vi "Test Cryo-Con Read.vi"() -> ()   [LabVIEW 2016]
panel:
  out "data string":string
  out "Temperature":dbl format="%.5f"
  in  "VISA Resource Name":refnum<visa-resource-name>
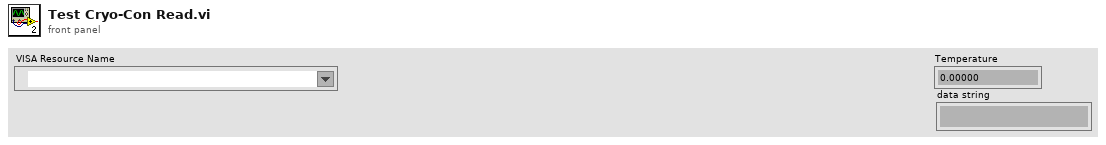
[diagram p1: front panel]
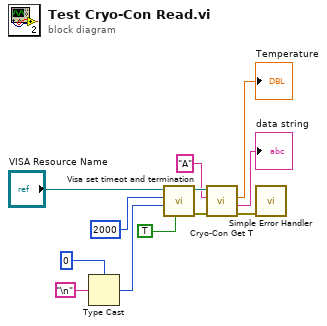
[diagram p0: block diagram]
diagram:
  n1 = Type Cast(type=u8 0, x="\n") -> (*(type *) &x=w3:u8)
  n2 = call "Visa set timeot and termination.vi"("Termination Character Enable"=TRUE, "Termination Character"=w3, "Timeout Value"=u32 2000, "VISA resource name"="VISA Resource Name") -> ("error out"=w2:errorcluster, "VISA resource name out"=w8:refnum<visa-resource-name>)  [unwired: 3 in, 3 out]
  n3 = call "Cryo-Con Get T.vi"("error in (no error)"=w2, "Channel"="A", "VISA Resource Name"=w8) -> ("error out"=w12:errorcluster, "data string"=→"data string":string, "Temperature"=→"Temperature":dbl)  [unwired: 5 in, 1 out]
  n4 = call <vilib>:"Simple Error Handler.vi"("error in (no error)"=w12) -> ()  [unwired: 4 in, 5 out]
